vi "Destruct Tag_By Ref.vi"(8 "error in (no error)":errorcluster, 10 "Tag Ref in":refnum<data-value>) -> (0 "error out":errorcluster, 2 "deleted":bool)   [LabVIEW 2020, in "Tag Engine.lvlib"]
doc: "Destruct a single Tag by reference.\n\nNo error is returned if the tag is not found."
uses:
  Tag Engine.lvlib
  Tag/Tag.lvclass
  Core/Tag Core.lvclass
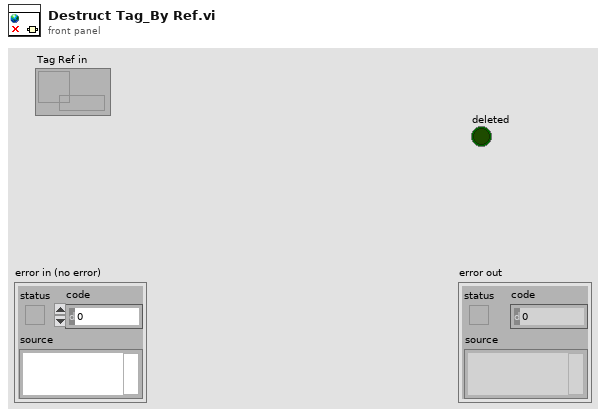
[diagram p1: front panel]
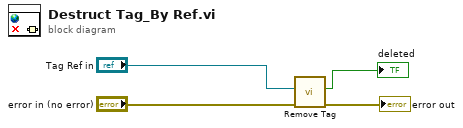
[diagram p0: block diagram]
diagram:
  n1 = call "Remove Tag.vi"("error in (no error)"="error in (no error)", "Tag Reference in"="Tag Ref in") -> ("error out"=→"error out":errorcluster, "removed?"=→"deleted":bool)  [unwired: 8 in]
